vi "DAQ Assist Output 2.vi"(7 "index":i32) -> ()   [LabVIEW 2015]
panel:
  in  "data":u32[](array[numeric])=[128, 144, 192, 160, 161, 162, 163, 164, 165, 166, 167, 168]
  out "error out":errorcluster
  in  "device name":tag="Dev2"
  in  "error in":errorcluster
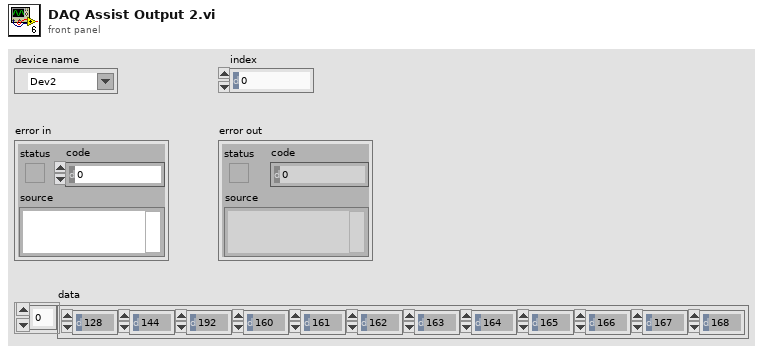
[diagram p1: front panel]
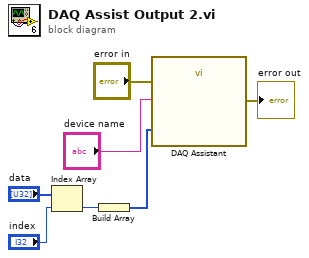
[diagram p0: block diagram]
diagram:
  n1 = Index Array(array="data", index="index") -> (element=w2:u32)
  n2 = Build Array(w2) -> (w1:u32[])
  n3 = call "DAQ Assistant"("data"=w1, "error in"="error in", "device name"="device name") -> ("error out"=→"error out":errorcluster)  [unwired: 15 in, 1 out]
